vi "AnalyseLaserResponse.vi"(8 "error in (no error)":errorcluster, 9 "Power":dbl[](array[numeric]), 10 "Constrol":u32[](array[numeric]), 11 "HC-LaserPulse in":refnum<class "HC-LaserResponse.lvclass">) -> (0 "error out":errorcluster, 2 "Results":T1, 3 "HC-LaserPulse out":refnum<class "HC-LaserResponse.lvclass">)   [LabVIEW 2013, in "HardwareCharacterization.lvlib" / "HC-LaserResponse.lvclass"]
uses:
  HC-LaserResponse.lvclass
  Test-results.ctl
  HC-LaserResponse.lvclass/HC-LaserResponse.ctl
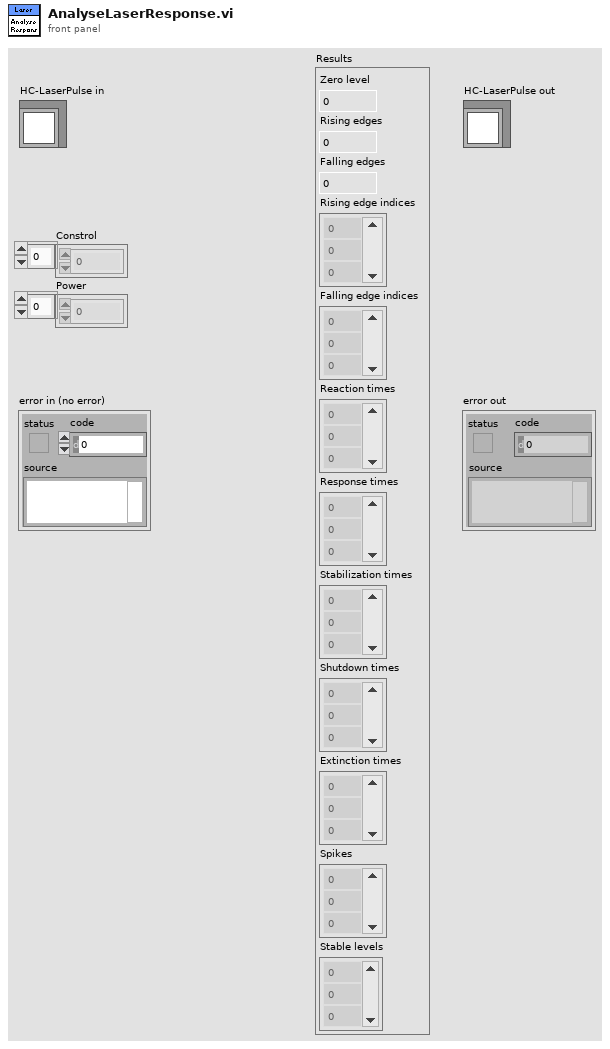
[diagram p1: front panel]
types:
  T1 = typedef "HardwareCharacterization.lvlib/HC-LaserResponse.lvclass/Test-results.ctl" = cluster{"Zero level":dbl, "Rising edges":i32, "Falling edges":i32, "Rising edge indices":dbl[], "Falling edge indices":dbl[], "Reaction times":dbl[], "Response times":dbl[], "Stabilization times":dbl[], "Shutdown times":dbl[], "Extinction times":dbl[], "Spikes":i32[], "Stable levels":dbl[]}
  T2 = typedef "HardwareCharacterization.lvlib/HC-LaserResponse.lvclass/Settings-extinction.ctl" = cluster{"Treshold [%]":i32}
  T3 = typedef "HardwareCharacterization.lvlib/HC-LaserResponse.lvclass/Settings-shutdown.ctl" = cluster{"Treshold [%]":i32}
  T4 = typedef "HardwareCharacterization.lvlib/HC-LaserResponse.lvclass/Settings-stabilization.ctl" = cluster{"Max. delta [%]":i32, "Min. segment length":i32}
  T5 = typedef "HardwareCharacterization.lvlib/HC-LaserResponse.lvclass/Settings-response.ctl" = cluster{"Treshold [%]":i32}
  T6 = typedef "HardwareCharacterization.lvlib/HC-LaserResponse.lvclass/Test-characteristics.ctl" = cluster{"Record length":i32, "Time interval [s]":dbl, "Note":string, "Laser control mode":enum16{"Undefined", "Modulation (digital)", "Power variation (analog)"}, "Power [Watt]":dbl, "Power [%]":dbl, "Pulse rate [Hz]":dbl, "Detector":T7, "Duty cycle [%]":dbl}
  T7 = typedef "HardwareCharacterization.lvlib/HC-LaserResponse.lvclass/Detectors.ctl" = enum16{"Undefined", "DET10A", "DET10A - 2kOhm ", "PDA36A - 0dB"}
  T8 = typedef "HardwareCharacterization.lvlib/HC-LaserResponse.lvclass/Settings-reaction.ctl" = cluster{"Treshold [%]":i32}
  T9 = typedef "HardwareCharacterization.lvlib/HC-LaserResponse.lvclass/Settings-stable.ctl" = cluster{"Top fraction [%]":i32, "Max. delta [Volt]":dbl, "Min. segment length":i32}
  T10 = typedef "HardwareCharacterization.lvlib/HC-LaserResponse.lvclass/Settings-zero.ctl" = cluster{"Lower fraction [%]":i32, "Max. delta [Volt]":dbl, "Min. segment length":i32}
  T11 = typedef "HardwareCharacterization.lvlib/HC-LaserResponse.lvclass/Settings-divide.ctl" = cluster{"Accept only complete pulses":bool, "Edge treshold [%]":i32}
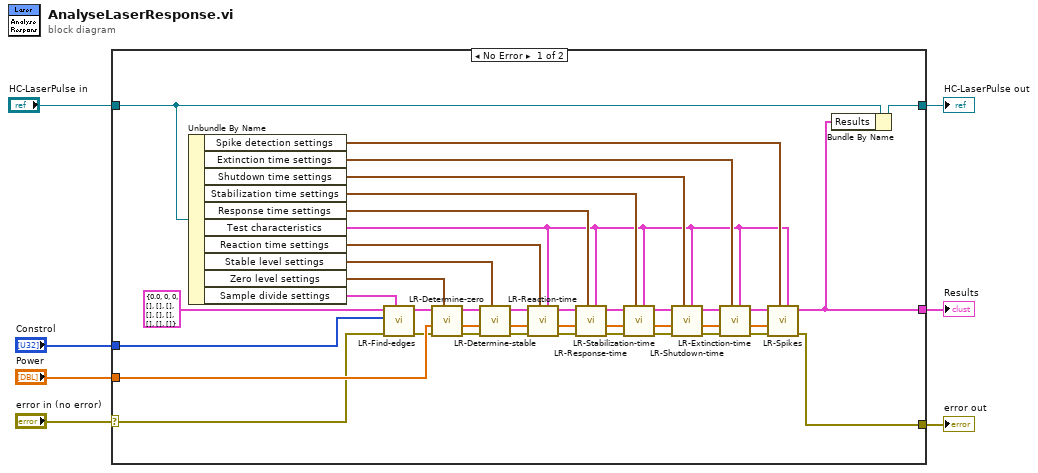
[diagram p0: block diagram]
diagram:
  n1 = case shown="No Error" "error in (no error)" {
    selector: "error in (no error)" -> [w9 w50]
    tunnel: [w22 w50] -> w6
    tunnel: [w19 w49] -> w4
    tunnel: "HC-LaserPulse in" -> [w48 w49]
    tunnel: "Constrol" -> [w10 _]
    tunnel: "Power" -> [w11 _]
    tunnel: [w18 _] -> w1
    frame No Error {
      n2 = Unbundle By Name(w48) -> ("Spike detection settings"=w21:cluster{"Treshold [%]":i32}, "Extinction time settings"=w26:T2, "Shutdown time settings"=w32:T3, "Stabilization time settings"=w37:T4, "Response time settings"=w38:T5, "Test characteristics"=w20:T6, "Reaction time settings"=w42:T8, "Stable level settings"=w44:T9, "Zero level settings"=w45:T10, "Sample divide settings"=w14:T11)
      n3 = call "LR-Find-edges.vi"("Sample divide settings"=w14, "error in (no error)"=w9, "Control in"=w10, "Results in"=T1 {"Zero level"=0.0, "Rising edges"=0, "Falling edges"=0, "Rising edge indices"=[], "Falling edge indices"=[], "Reaction times"=[], "Response times"=[], "Stabilization times"=[], "Shutdown times"=[], "Extinction times"=[], "Spikes"=[], "Stable levels"=[]} ("Results")) -> ("error out"=w8:errorcluster, "Results"=w12:T1)  [unwired: 4 in, 2 out]
      n4 = call "LR-Determine-zero.vi"("Zero level settings"=w45, "error in (no error)"=w8, "Power in"=w11, "Results in"=w12) -> ("error out"=w46:errorcluster, "Power"=w47:dbl[], "Results"=w43:T1)  [unwired: 4 in, 1 out]
      n5 = call "LR-Determine-stable.vi"("Stable level settings"=w44, "error in (no error)"=w46, "Power in"=w47, "Results in"=w43) -> ("error out"=w16:errorcluster, "Power"=w17:dbl[], "Results"=w15:T1)  [unwired: 4 in, 1 out]
      n6 = call "LR-Reaction-time.vi"("Test characteristics"=w20, "Reaction time settings"=w42, "error in (no error)"=w16, "Power in"=w17, "Results in"=w15) -> ("error out"=w39:errorcluster, "Power"=w40:dbl[], "Results"=w41:T1)  [unwired: 3 in, 1 out]
      n7 = call "LR-Response-time.vi"("Test characteristics"=w20, "Response time settings"=w38, "error in (no error)"=w39, "Power in"=w40, "Results in"=w41) -> ("error out"=w35:errorcluster, "Power"=w34:dbl[], "Results"=w36:T1)  [unwired: 3 in, 1 out]
      n8 = call "LR-Stabilization-time.vi"("Test characteristics"=w20, "Stabilization time settings"=w37, "error in (no error)"=w35, "Power in"=w34, "Results in"=w36) -> ("error out"=w30:errorcluster, "Power"=w31:dbl[], "Results"=w33:T1)  [unwired: 3 in, 1 out]
      n9 = call "LR-Shutdown-time.vi"("Test characteristics"=w20, "Shutdown time settings"=w32, "error in (no error)"=w30, "Power in"=w31, "Results in"=w33) -> ("error out"=w27:errorcluster, "Power"=w28:dbl[], "Results"=w29:T1)  [unwired: 3 in, 1 out]
      n10 = call "LR-Extinction-time.vi"("Test characteristics"=w20, "Extinction time settings"=w26, "error in (no error)"=w27, "Power in"=w28, "Results in"=w29) -> ("error out"=w23:errorcluster, "Power"=w24:dbl[], "Results"=w25:T1)  [unwired: 3 in, 1 out]
      n11 = call "LR-Spikes.vi"("Test characteristics"=w20, "Spike detection settings"=w21, "error in (no error)"=w23, "Power in"=w24, "Results in"=w25) -> ("error out"=w22:errorcluster, "Results"=w18:T1)  [unwired: 3 in, 2 out]
      n12 = Bundle By Name(cluster=w48, "Results"=w18) -> (w19:refnum<class "HC-LaserResponse.lvclass">)
    }
    frame Error {
    }
  }
  "error out" <- w6
  "HC-LaserPulse out" <- w4
  "Results" <- w1
